vi "Execution End.vi"(8 "error in (no error)":errorcluster, 10 "Execution in":refnum<data-value>, 11 "CsvReportPlugin in":refnum<class "CsvReportPlugin.lvclass">) -> (0 "error out":errorcluster, 2 "Execution out":refnum<data-value>, 3 "CsvReportPlugin out":refnum<class "CsvReportPlugin.lvclass">)   [LabVIEW 2015, in "CsvReportPlugin.lvclass"]
uses:
  CsvReportPlugin.lvclass
  Core/Execution.lvclass
  Core/Execution/EXECUTION_RESULT_TYPEDEF.ctl
  Core/Project.lvclass
  Core/Step.lvclass
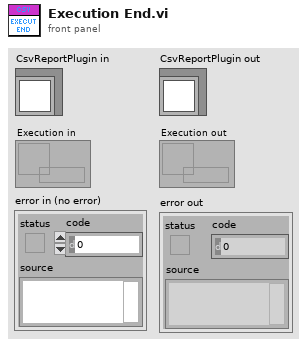
[diagram p1: front panel]
types:
  T1 = typedef "Execution.lvclass/EXECUTION_RESULT_TYPEDEF.ctl" = enum16{"Unknow", "Terminated", "Passed", "Failed", "Error"}
  T2 = typedef "Execution.lvclass/EXECUTION_CONTEXT.ctl" = cluster{"Continue Test":bool, "DUT Info":T3, "StartTime":timestamp, "EndTime":timestamp, "Result":T1, "Info Text":string, "ResultList":T4[]}
  T3 = typedef "Execution.lvclass/DUT_INFO_TYPEDEF.ctl" = cluster{"SN":string, "Model":string, "PartNumber":string, "Revision":string, "Software":string, "Hardware":string}
  T4 = typedef "Execution.lvclass/STEP_RESULT.ctl" = cluster{"StepIndex":u32, "Step":refnum<class "Step.lvclass">, "StartTime":timestamp, "EndTime":timestamp, "Result":T5, "Error Info":string, "Measure Results":T6[]}
  T5 = typedef "Step.lvclass/STEP_STATUS.ctl" = enum16{"Skipped", "Done", "Passed", "Failed", "Error"}
  T6 = typedef "Execution.lvclass/STEP_MEASURE_RESULT.ctl" = cluster{"Name":string, "Data Type":T7, "Check Type":T8, "String Limit":string, "Lower Limit":dbl, "Upper Limit":dbl, "Boolean Limit":bool, "Ignore Case":bool, "Measure Data":variant, "Result":T5, "Error Info":string}
  T7 = typedef "Step.lvclass/OUTPUT_DATA_TYPE.ctl" = enum16{"Boolean", "String", "Numeric", "Other"}
  T8 = typedef "Step.lvclass/OUTPUT_CHECK_TYPE.ctl" = enum16{"INVALID", "DO_NOT_CHECK", "RECORD", "VARIABLE", "EQUAL", "NOT_EQUAL", "STR_CONTAINS", "STR_START_WITH", "STR_END_WITH", "STR_REGEX_MATCH", "NUM_GT", "NUM_LT", "NUM_GE", "NUM_LE", "NUM_RANGE", "NUM_RANGE_BDY"}
  T9 = enum16{"open", "replace", "create", "open or create", "replace or create", "replace or create with confirmation"}
  T10 = typedef "STATION_INFO_TYPEDEF.ctl" = cluster{"Process":string, "Station Name":string, "Fixture":string, "Production Line":string, "Factory":string}
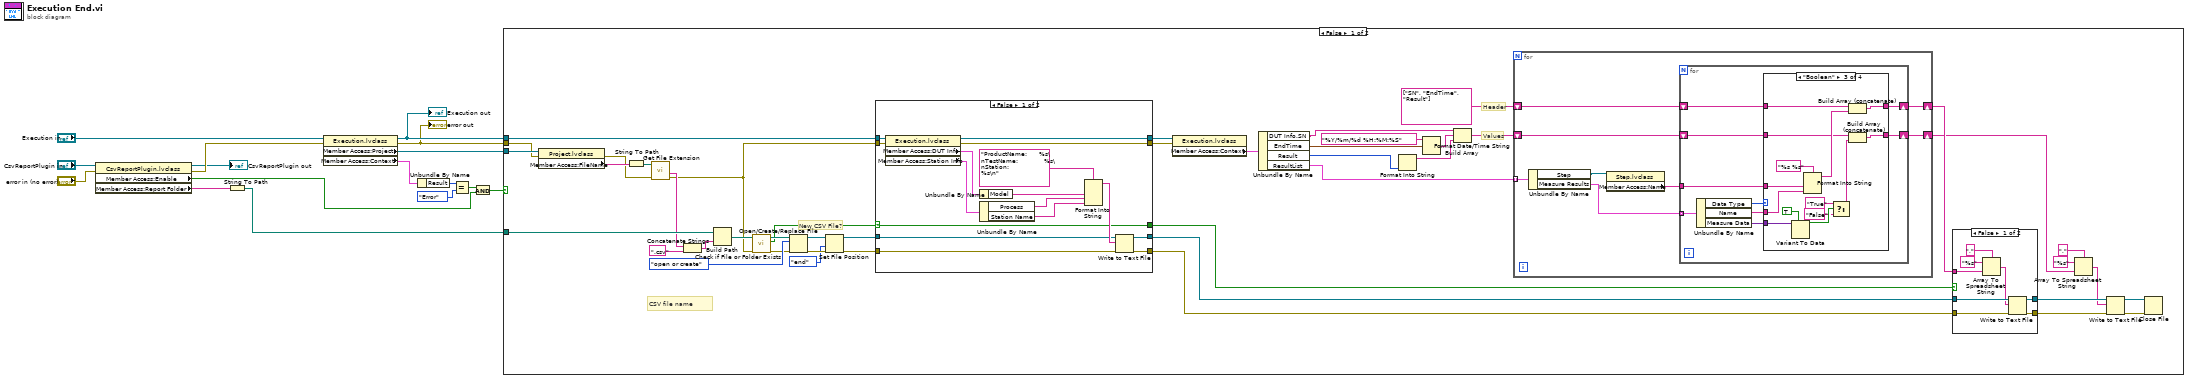
[diagram p0: block diagram]
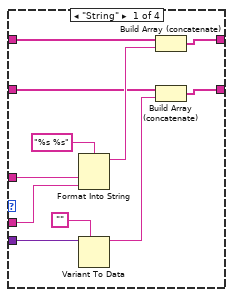
[diagram p3: hidden frame]
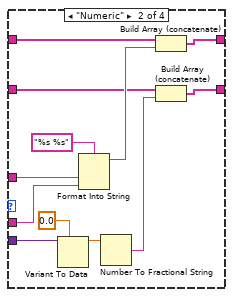
[diagram p4: hidden frame]
diagram:
  n1 = property class="CsvReportPlugin.lvclass"(reference="CsvReportPlugin in", error in="error in (no error)") -> (reference out=→"CsvReportPlugin out":refnum<class "CsvReportPlugin.lvclass">, error out=w12:errorcluster, "Member Access:Enable"=w4:bool, "Member Access:Report Folder"=w5:string)
  n2 = String To Path(string=w5) -> (path=w10:path)
  n3 = property class="Execution.lvclass"(reference="Execution in", error in=w12) -> (reference out=w3:refnum<data-value>, error out=w2:errorcluster, "Member Access:Project"=w14:refnum<class "Project.lvclass">, "Member Access:Context"=w9:T2)
  "error out" <- w2
  "Execution out" <- w3
  n4 = Unbundle By Name(w9) -> ("Result"=w8:T1)
  n5 = Equal?(x=w8, y=EXECUTION_RESULT_TYPEDEF."Error") -> (x = y?=w6:bool)
  n6 = And(x=w6, y=w4) -> (x .and. y?=w1:bool)
  n7 = case shown="False" w1 {
    tunnel: w14 -> [w61 _]
    tunnel: w2 -> [w59 _]
    tunnel: w10 -> [w56 _]
    tunnel: w3 -> [w51 _]
    frame False {
      # "Values"
      # "Header"
      # "New CSV File?"
      # "CSV file name"
      n8 = property class="Project.lvclass"(reference=w61, error in=w59) -> (error out=w57:errorcluster, "Member Access:FileName"=w60:string)  [unwired: 1 out]
      n9 = String To Path(string=w60) -> (path=w58:path)
      n10 = call <vilib>:"Get File Extension.vi"("error in (no error)"=w57, "file"=w58) -> ("error out"=w44:errorcluster, "filename without extension"=w55:string)  [unwired: 5 in, 3 out]
      n11 = Concatenate Strings(w55, ".csv") -> (w54:string)
      n12 = Build Path(base path=w56, name or relative path=w54) -> (appended path=w52:path)
      n13 = call <vilib>:"Check if File or Folder Exists.vi"("error in (no error)"=w44, "path"=w52) -> ("error out"=w45:errorcluster, "file or folder exists?"=w43:bool, "dup path"=w46:path)  [unwired: 7 in]
      n14 = Open/Create/Replace File(file path (use dialog)=w46, error in=w45, operation (0:open)=T9."open or create") -> (refnum out=w48:refnum<file>, error out=w50:errorcluster)  [unwired: 3 in, 1 out]
      n15 = Set File Position(refnum=w48, from (0:start)=enum16{"start", "end", "current"}."end", error in=w50) -> (refnum out=w42:refnum<file>, error out=w41:errorcluster)  [unwired: 1 in]
      n16 = case shown="False" w43 {
        selector: w43 -> [w129 w145]
        tunnel: w51 -> [w143 w148]
        tunnel: w44 -> [w142 w144]
        tunnel: w42 -> [w134 w146]
        tunnel: w41 -> [w133 w147]
        tunnel: [w132 w146] -> w27
        tunnel: [w131 w147] -> w28
        tunnel: [w130 w148] -> w40
        tunnel: [w129 w145] -> w26
        tunnel: [w128 w144] -> w32
        frame False {
          n17 = property class="Execution.lvclass"(reference=w143, error in=w142) -> (reference out=w130:refnum<data-value>, error out=w128:errorcluster, "Member Access:DUT Info"=w140:T3, "Member Access:Station Info"=w139:T10)
          n18 = Unbundle By Name(w140) -> ("Model"=w138:string)
          n19 = Unbundle By Name(w139) -> ("Process"=w137:string, "Station Name"=w136:string)
          n20 = Format Into String(format string="ProductName:      %s\nTestName:             %s\nStation:                   %s\n", w138, w137, w136) -> (resulting string=w135:string)  [unwired: 2 in, 1 out]
          n21 = Write to Text File(file (use dialog)=w134, text=w135, error in=w133) -> (refnum out=w132:refnum<file>, error out=w131:errorcluster)  [unwired: 1 in, 1 out]
        }
        frame True {
        }
      }
      n22 = property class="Execution.lvclass"(reference=w40, error in=w32) -> ("Member Access:Context"=w39:T2)  [unwired: 2 out]
      n23 = Unbundle By Name(w39) -> ("DUT Info.SN"=w35:string, "EndTime"=w37:timestamp, "Result"=w36:T1, "ResultList"=w31:T4[])
      n24 = Format Into String(w36) -> (resulting string=w33:string)  [unwired: 3 in, 1 out]
      n25 = Format Date/Time String(time format string (%c)="%Y/%m/%d %H:%M:%S", seconds (now)=w37) -> (date/time string=w34:string)  [unwired: 1 in]
      n26 = Build Array(w35, w34, w33) -> (w29:string[])
      n27 = for {
        tunnel: w31 -> [w77] mode=indexing
        shift-right: [w73] -> w25
        shift-left: string[] ["SN", "EndTime", "Result"] -> [w79]
        shift-right: [w72] -> w20
        shift-left: w29 -> [w78]
        n28 = Unbundle By Name(w77) -> ("Step"=w76:refnum<class "Step.lvclass">, "Measure Results"=w75:T6[])
        n29 = property class="Step.lvclass"(reference=w76) -> ("Member Access:Name"=w74:string)  [unwired: 1 in, 2 out]
        n30 = for {
          shift-right: [w80] -> w72
          shift-left: w78 -> [w82]
          shift-right: [w81] -> w73
          shift-left: w79 -> [w83]
          tunnel: w75 -> [w87] mode=indexing
          tunnel: w74 -> [w88]
          n31 = Unbundle By Name(w87) -> ("Data Type"=w86:T7, "Name"=w85:string, "Measure Data"=w84:variant)
          n32 = case shown="\"Boolean\"" w86 {
            tunnel: w88 -> [w98 w110 w124 _]
            tunnel: w85 -> [w97 w109 w123 _]
            tunnel: w84 -> [w96 w108 w122 _]
            tunnel: w83 -> [w94 w106 w120 w127]
            tunnel: w82 -> [w92 w104 w118 w126]
            tunnel: [w90 w103 w117 w127] -> w81
            tunnel: [w89 w102 w116 w126] -> w80
            frame "String" {
              n33 = Format Into String(format string="%s %s", w98, w97) -> (resulting string=w93:string)  [unwired: 2 in, 1 out]
              n34 = Variant To Data(type="", Variant=w96) -> (data=w91:string)  [unwired: 1 in, 1 out]
              n35 = Build Array (concatenate)(w94, w93) -> (w90:string[])
              n36 = Build Array (concatenate)(w92, w91) -> (w89:string[])
            }
            frame "Numeric" {
              n37 = Variant To Data(type=0.0, Variant=w108) -> (data=w101:dbl)  [unwired: 1 in, 1 out]
              n38 = Format Into String(format string="%s %s", w110, w109) -> (resulting string=w105:string)  [unwired: 2 in, 1 out]
              n39 = Number To Fractional String(number=w101) -> (F-format string=w100:string)  [unwired: 3 in]
              n40 = Build Array (concatenate)(w106, w105) -> (w103:string[])
              n41 = Build Array (concatenate)(w104, w100) -> (w102:string[])
            }
            frame "Boolean" {
              n42 = Variant To Data(type=TRUE, Variant=w122) -> (data=w115:bool)  [unwired: 1 in, 1 out]
              n43 = Format Into String(format string="%s %s", w124, w123) -> (resulting string=w119:string)  [unwired: 2 in, 1 out]
              n44 = Select(t="True", s=w115, f="False") -> (s? t:f=w112:string)
              n45 = Build Array (concatenate)(w120, w119) -> (w117:string[])
              n46 = Build Array (concatenate)(w118, w112) -> (w116:string[])
            }
            frame "Other" {
            }
          }
        }
      }
      n47 = case shown="False" w26 {
        tunnel: w28 -> [w69 w70]
        tunnel: w27 -> [w68 w71]
        tunnel: w25 -> [w67 _]
        tunnel: [w64 w71] -> w24
        tunnel: [w63 w70] -> w23
        frame False {
          n48 = Array To Spreadsheet String(delimiter (Tab)=",", array=w67, 3:"%s") -> (spreadsheet string=w62:string)
          n49 = Write to Text File(file (use dialog)=w68, text=w62, error in=w69) -> (refnum out=w64:refnum<file>, error out=w63:errorcluster)  [unwired: 1 in, 1 out]
        }
        frame True {
        }
      }
      n50 = Array To Spreadsheet String(delimiter (Tab)=",", array=w20, 3:"%s") -> (spreadsheet string=w17:string)
      n51 = Write to Text File(file (use dialog)=w24, text=w17, error in=w23) -> (refnum out=w19:refnum<file>, error out=w18:errorcluster)  [unwired: 1 in, 1 out]
      n52 = Close File(refnum=w19, error in=w18) -> ()  [unwired: 2 out]
    }
    frame True {
    }
  }
